vi "resistance2color.vi"() -> (5 "Finish":bool, 6 "Correct or not?":bool, 7 "Answear Time (sec)":dbl)   [LabVIEW 2014]
uses:
  Colors.ctl
panel:
  out "Question":dbl
  out "Band 3":u32(colorbox)=16750592
  out "Band 2":u32(colorbox)=16067327
  out "Band 1":u32(colorbox)=16776960
  out "finish time":u32
  out "start time":u32
  out "Your Guess":dbl
  in  "Color Band 3":T1=11 items=["Black"=0, "Brown"=1, "Red"=2, "Orange"=3, "Yellow"=4, "Green"=5, "Blue"=6, "Purple"=7, "Grey"=8, "White"=9, "Please Select"=11]
  in  "Color Band 1":T1=11 items=["Black"=0, "Brown"=1, "Red"=2, "Orange"=3, "Yellow"=4, "Green"=5, "Blue"=6, "Purple"=7, "Grey"=8, "White"=9, "Please Select"=11]
  in  "Color Band 2":T1=11 items=["Black"=0, "Brown"=1, "Red"=2, "Orange"=3, "Yellow"=4, "Green"=5, "Blue"=6, "Purple"=7, "Grey"=8, "White"=9, "Please Select"=11]
  out "Invalid Color":bool
  out "Resistor Value":dbl
  in  "OK":bool
  # "Plaease choose the \"Color Band {1,2,3}\" properly,\nso that the resistance is exactly:"
  # "(Ohm)"
  # "(Ohm)"
  # "(-1 means invalid resistance, e.g. color band 1 is black OR some band weren't selected)"
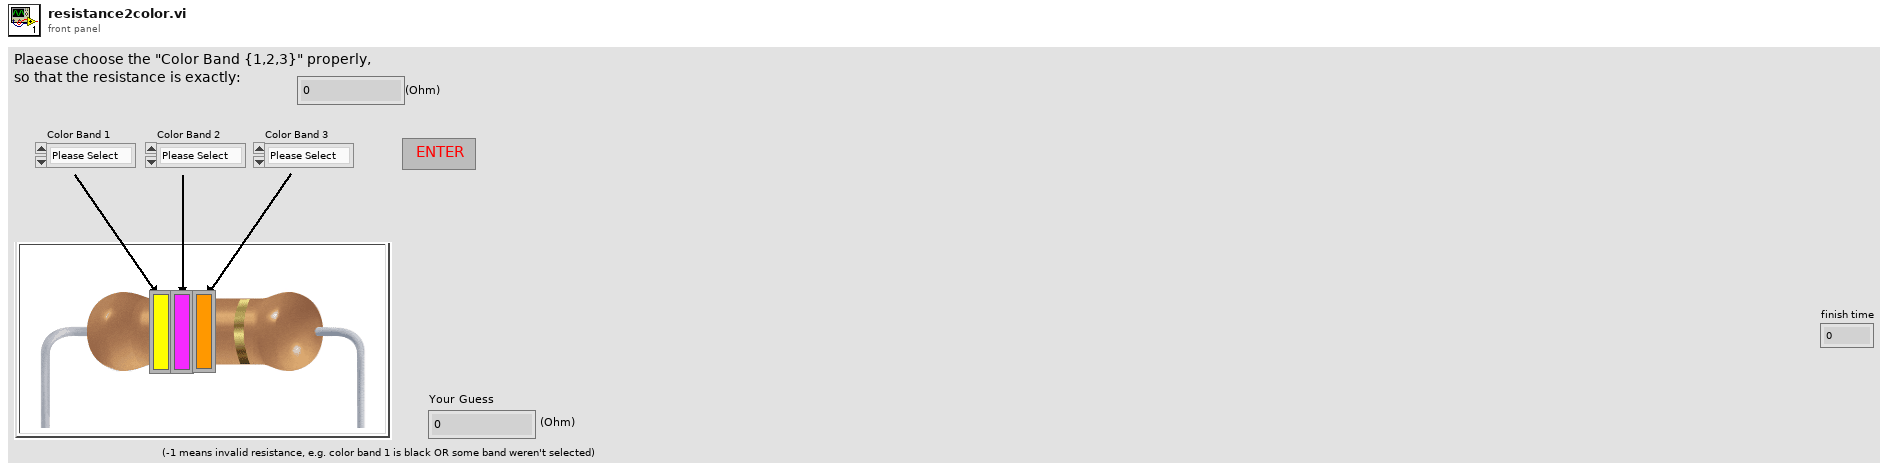
[diagram p1: front panel]
types:
  T1 = typedef "Colors.ctl" = u16
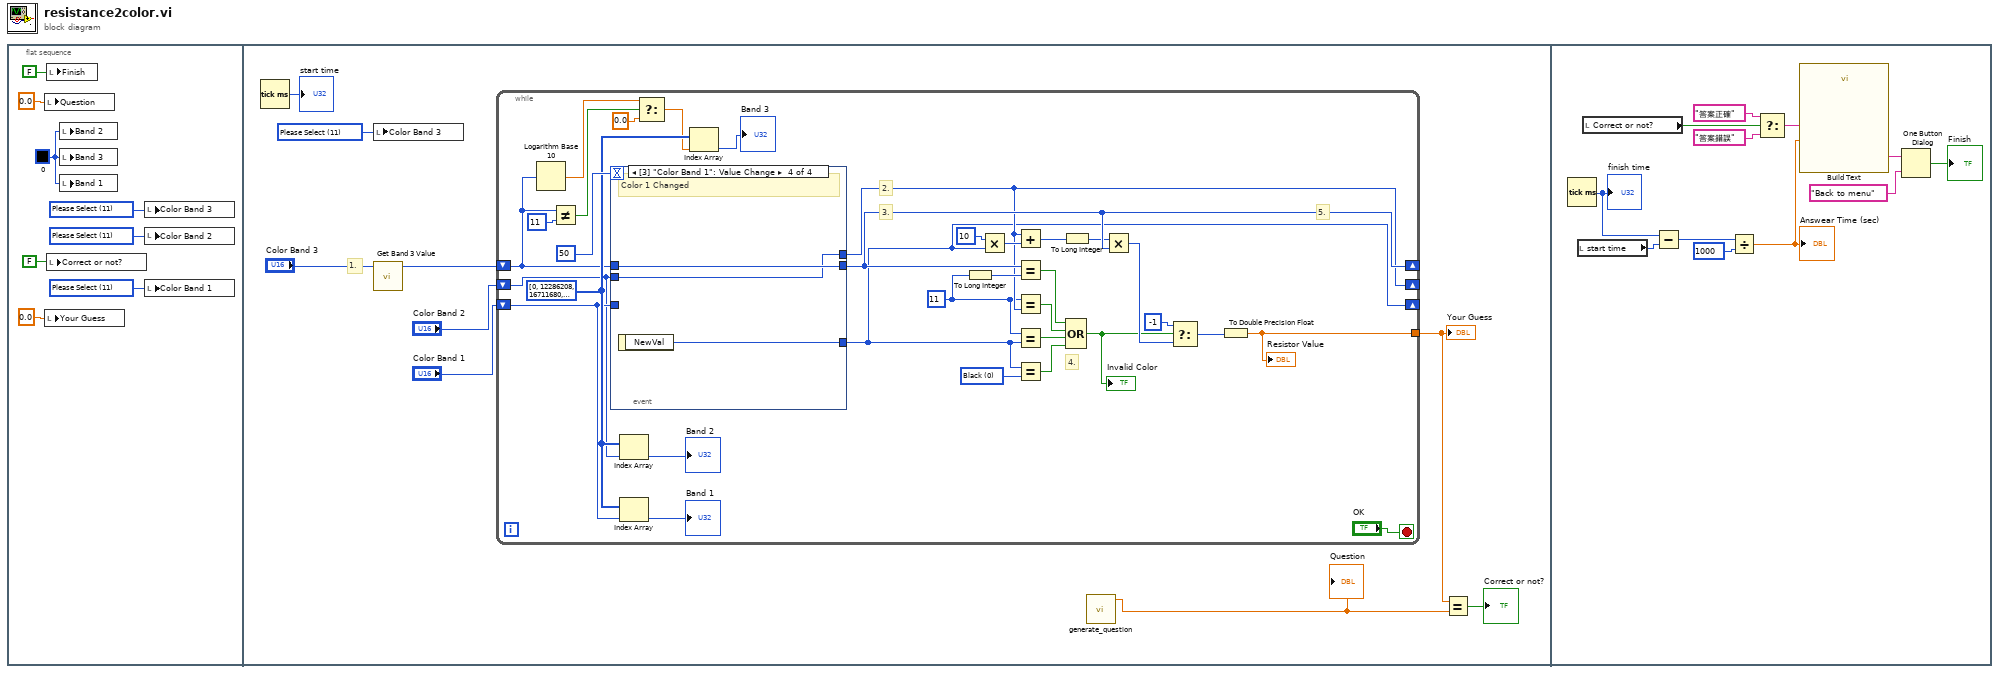
[diagram p0: block diagram]
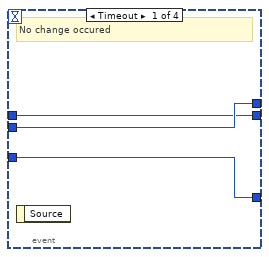
[diagram p2: hidden frame]
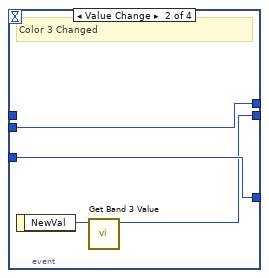
[diagram p3: hidden frame]
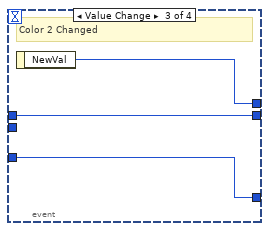
[diagram p4: hidden frame]
diagram:
  n1 = flat-sequence {
    frame #0 {
      w2 = u32 0 ("Band 1")
      w4 = T1 11 items=["Black"=0, "Brown"=1, "Red"=2, "Orange"=3, "Yellow"=4, "Green"=5, "Blue"=6, "Purple"=7, "Grey"=8, "White"=9, "Please Select"=11] ("Color Band 3")
      w5 = T1 11 items=["Black"=0, "Brown"=1, "Red"=2, "Orange"=3, "Yellow"=4, "Green"=5, "Blue"=6, "Purple"=7, "Grey"=8, "White"=9, "Please Select"=11] ("Color Band 3")
      w6 = T1 11 items=["Black"=0, "Brown"=1, "Red"=2, "Orange"=3, "Yellow"=4, "Green"=5, "Blue"=6, "Purple"=7, "Grey"=8, "White"=9, "Please Select"=11] ("Color Band 3")
      n2 = local write "Question"(0.0 ("number 2")) -> ()
      n3 = local write "Your Guess"(0.0 ("Question 4")) -> ()
      n4 = local write "Finish"(FALSE ("Finish 2")) -> ()
      n5 = local write "Correct or not?"(FALSE ("Correct or not?")) -> ()
      n6 = local write "Band 2"(w2) -> ()
      n7 = local write "Band 3"(w2) -> ()
      n8 = local write "Band 1"(w2) -> ()
      n9 = local write "Color Band 3"(w5) -> ()
      n10 = local write "Color Band 2"(w4) -> ()
      n11 = local write "Color Band 1"(w6) -> ()
    }
    frame #1 {
      w11 = T1 11 items=["Black"=0, "Brown"=1, "Red"=2, "Orange"=3, "Yellow"=4, "Green"=5, "Blue"=6, "Purple"=7, "Grey"=8, "White"=9, "Please Select"=11] ("Color Band 3")
      # "1."
      n12 = Tick Count (ms)() -> (millisecond timer value=→"start time":u32)
      n13 = local write "Color Band 3"(w11) -> ()
      n14 = call "Get Band 3 Value.vi"("Color Band 3"="Color Band 3") -> ("Multiplier"=w17:i32)  [unwired: 10 in]
      n15 = while {
        shift-right: [w31] -> _
        shift-left: "Color Band 1" -> [w28]
        shift-right: [w37] -> _
        shift-left: "Color Band 2" -> [w27]
        shift-right: [w43] -> _
        shift-left: w17 -> [w23]
        tunnel: [w30] -> w14
        stop <- "OK" stop-if-true
        w29 = u32[] [0, 12286208, 16711680, 16750592, 16776960, 6618880, 3381759, 16067327, 11776947, 16448250] ("Resistor Colors")
        w33 = T1 0 items=["Black"=0, "Brown"=1, "Red"=2, "Orange"=3, "Yellow"=4, "Green"=5, "Blue"=6, "Violet"=7, "Grey"=8, "White"=9, "Please Select"=11] ("y")
        w35 = u16 11 ("y")
        # "5."
        # "4."
        # "3."
        # "2."
        # "Main Loop"
        n16 = Logarithm Base 10(1:w23) -> (0:w20:dbl)
        n17 = Not Equal?(x=w23, y=11) -> (x != y?=w21:bool)
        n18 = event shown="[3] \"Color Band 1\": Value Change" {
          selector: _ -> [_ _ _ _]
          dyn-events: _ -> [_ _ _ _]
          timeout: 50 -> [_ _ _ _]
          tunnel: [w53 w56 w59 w61] -> w31
          tunnel: [w52 w57 w58 w62] -> w37
          tunnel: [w51 w55 w60 w63] -> w43
          tunnel: w28 -> [w53 w56 w59 _]
          tunnel: w27 -> [w52 w57 _ w62]
          tunnel: w23 -> [w51 _ w60 w63]
          event Timeout {
            # "No change occured"
            n19 = event-data() -> ()  [unwired: 1 in, 1 out]
          }
          event Value Change {
            # "Color 3 Changed"
            n20 = event-data() -> ("NewVal"=w54:T1)  [unwired: 1 in]
            n21 = call "Get Band 3 Value.vi"("Color Band 3"=w54) -> ("Multiplier"=w55:i32)  [unwired: 10 in]
          }
          event Value Change {
            # "Color 2 Changed"
            n22 = event-data() -> ("NewVal"=w58:T1)  [unwired: 1 in]
          }
          event Value Change {
            # "Color 1 Changed"
            n23 = event-data() -> ("NewVal"=w61:T1)  [unwired: 1 in]
          }
        }
        n24 = Index Array(array=w29, index=w27) -> (element=→"Band 2":u32)
        n25 = Index Array(array=w29, index=w28) -> (element=→"Band 1":u32)
        n26 = Select(t=w20, s=w21, f=0.0) -> (s? t:f=w18:dbl)
        n27 = Index Array(array=w29, index=w18) -> (element=→"Band 3":u32)
        n28 = To Long Integer(number=w35) -> (32bit integer=w38:i32)
        n29 = Multiply(x=u16 10 ("y"), y=w31) -> (x*y=w50:T1)
        n30 = Add(x=w37, y=w50) -> (x+y=w40:T1)
        n31 = Equal?(x=w43, y=w38) -> (x = y?=w41:bool)
        n32 = Equal?(x=w35, y=w37) -> (x = y?=w42:bool)
        n33 = Equal?(x=w35, y=w31) -> (x = y?=w34:bool)
        n34 = Equal?(x=w31, y=w33) -> (x = y?=w32:bool)
        n35 = To Long Integer(number=w40) -> (32bit integer=w39:i32)
        n36 = Compound Arithmetic op=OR(w41, w42, w34, w32) -> (w44:bool)
        "Invalid Color" <- w44
        n37 = Multiply(x=w39, y=w43) -> (x*y=w47:i32)
        n38 = Select(t=-1, s=w44, f=w47) -> (s? t:f=w46:i32)
        n39 = To Double Precision Float(number=w46) -> (double precision float=w30:dbl)
        "Resistor Value" <- w30
      }
      "Your Guess" <- w14
      n40 = call "generate_question.vi"() -> ("Question"=w9:dbl)  [unwired: 11 in]
      "Question" <- w9
      n41 = Equal?(x=w14, y=w9) -> (x = y?=→"Correct or not?":bool)
    }
    frame #2 {
      n42 = Tick Count (ms)() -> (millisecond timer value=w75:u32)
      "finish time" <- w75
      n43 = local read "start time"() -> (w74:u32)
      n44 = local read "Correct or not?"() -> (w69:bool)
      n45 = Subtract(x=w75, y=w74) -> (x-y=w73:u32)
      n46 = Divide(x=w73, y=u32 1000) -> (x/y=w67:dbl)
      "Answear Time (sec)" <- w67
      n47 = Select(t="答案正確", s=w69, f="答案錯誤") -> (s? t:f=w68:string)
      n48 = call "Build Text"("correct_str"=w68, "ans_time"=w67) -> ("Result"=w66:string)  [unwired: 12 in, 1 out]
      n49 = One Button Dialog(message=w66, button name ("OK")="Back to menu") -> (true=→"Finish":bool)
    }
  }
